vi "putDataToQueueStateBoardvi.vi"(10 "STATE BOARD":T1, 11 "Queue in":refnum<queue>) -> ()   [LabVIEW 2017]
uses:
  controls/state_board_control.ctl
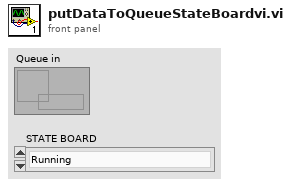
[diagram p1: front panel]
types:
  T1 = typedef "state_board_control.ctl" = enum16{"Running", "Waiting", "Pos", "IDLE"}
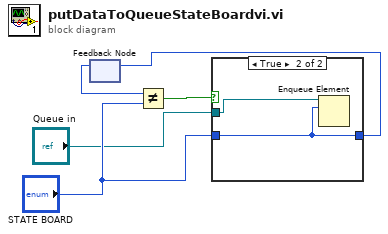
[diagram p0: block diagram]
diagram:
  n1 = feedback #1() -> (w5:T1)  [unwired: 1 in]
  n2 = Not Equal?(x=w5, y="STATE BOARD") -> (x != y?=w1:bool)
  n3 = case shown="True" w1 {
    tunnel: "STATE BOARD" -> [w6 w8]
    tunnel: [w6 w8] -> w4
    tunnel: "Queue in" -> [_ w7]
    frame False {
    }
    frame True {
      n4 = Enqueue Element(queue=w7, element=w8) -> ()  [unwired: 2 in, 3 out]
    }
  }
  n5 = feedback-in #1(w4) -> ()
